vi "ZCAN_OpenDevice.vi"(8 "error in (no error)":errorcluster caption="错误输入（无错误）", 9 "reserved":u32, 10 "device_index":u32, 11 "device_type":u32) -> (0 "error out":errorcluster caption="错误输出", 2 "DEVICE_HANDLE":u32)   [LabVIEW 2018]
doc: "该函数用于打开设备，一个设备只能被打开一次，返回值为设备句柄。\n注意：关闭程序前要调用ZCAN_CloseDevice释放设备句柄，否则第二次无法打开；\n\n如忘记释放句柄，需要关闭整个LabVIEW程序，CAN卡重新插拔。"
uses:
  zlgcan_labview_20220510/zlgcan_demo_DTU/bin/zlgcan_wrap.dll
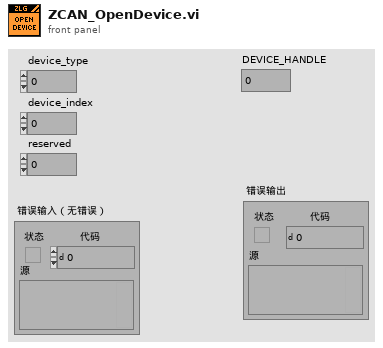
[diagram p1: front panel]
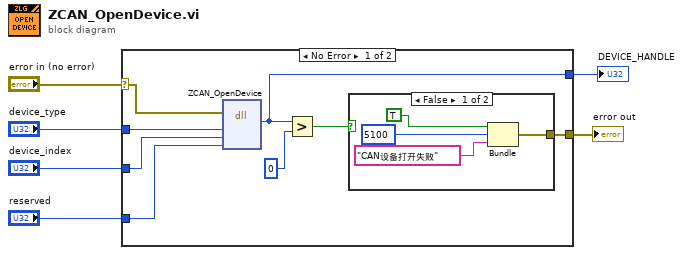
[diagram p0: block diagram]
diagram:
  n1 = case shown="No Error" "error in (no error)" {
    selector: "error in (no error)" -> [w10 w19]
    tunnel: [w8 w19] -> w5
    tunnel: "device_type" -> [w14 _]
    tunnel: "device_index" -> [w13 _]
    tunnel: "reserved" -> [w12 _]
    tunnel: [w7 _] -> w1
    frame No Error {
      n2 = dll-call lib="C:/Users/admin/Desktop/zlgcan_labview_20220510/zlgcan_demo_DTU/bin/zlgcan_wrap.dll" fn="ZCAN_OpenDevice"(error in=w10, "device_type"=w14, "device_index"=w13, "reserved"=w12) -> ("DEVICE_HANDLE"=w7:u32)  [unwired: 5 in, 2 out]
      n3 = Greater?(x=w7, y=u32 0) -> (0:w9:bool)
      n4 = case shown="False" w9 {
        tunnel: [w17 _] -> w8
        frame False {
          n5 = Bundle("status"=TRUE, "code"=5100, "消息"="CAN设备打开失败") -> (w17:cluster{"status":bool, "code":i32, "消息":string})  [unwired: 1 in]
        }
        frame True {
        }
      }
    }
    frame Error {
    }
  }
  "error out" <- w5
  "DEVICE_HANDLE" <- w1
